vi "Rodriguez_ExTask3_1-25-17.vi"() -> ()   [LabVIEW 2014, in "Rodriguez1_Visage_5th_LegoRobotics_11-29-16.lvrbt"]
uses:
  Rodriguez1_Visage_5th_LegoRobotics_11-29-16.lvrbt
panel:
  out "Random Number":dbl
  out "Moving Average":dbl
  in  "stop":bool
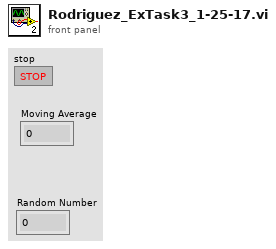
[diagram p1: front panel]
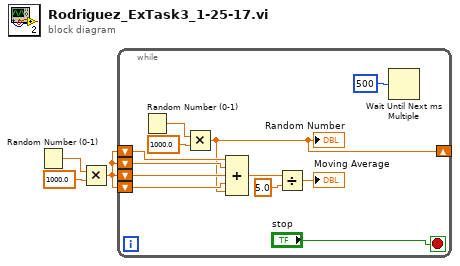
[diagram p0: block diagram]
diagram:
  n1 = Random Number (0-1)() -> (number: 0 to 1=w3:dbl)
  n2 = Multiply(x=w3, y=1000.0) -> (x*y=w1:dbl)
  n3 = while {
    shift-right: [w9] -> _
    shift-left: w1 -> [w10]
    shift-left: w1 -> [w12]
    shift-left: w1 -> [w13]
    shift-left: w1 -> [w11]
    stop <- "stop" stop-if-true
    n4 = Random Number (0-1)() -> (number: 0 to 1=w15:dbl)
    n5 = Multiply(x=w15, y=1000.0) -> (x*y=w9:dbl)
    "Random Number" <- w9
    n6 = Compound Arithmetic op=ADD(w10, w11, w12, w13, w9) -> (w8:dbl)
    n7 = Divide(x=w8, y=5.0) -> (x/y=→"Moving Average":dbl)
    n8 = Wait Until Next ms Multiple(millisecond multiple=u32 500) -> ()  [unwired: 1 out]
  }
